vi "AO Engine Testing.vi"(8 "error in (no error)":errorcluster) -> (0 "error out":errorcluster)   [LabVIEW 2009]
doc: "Copyright © 2005, Soliton Technologies.\nAll rights reserved."
uses:
  Controls/SLL DE List of Analog Outputs.ctl
  Controls/SLL DE AO Global Options.ctl
  <vilib>/DAQmx/read.llb/DAQmx Read (Analog DBL 1Chan 1Samp).vi
  <vilib>/DAQmx/create/channels.llb/DAQmx Create Channel (AI-Voltage-Basic).vi
panel:
  in  "stop":bool
  out "x-y":u32=6905
  out "Done?":bool
  out "data":dbl=0.000762939453125 format="%0.2f"
  in  "DAQmx Physical Channel":tag="Dev1/_ao0_vs_aognd"
  in  "AO Option":T1=enum."Write Line"
  in  "List of Analog Outputs":T2
  in  "AO value":dbl=1.0
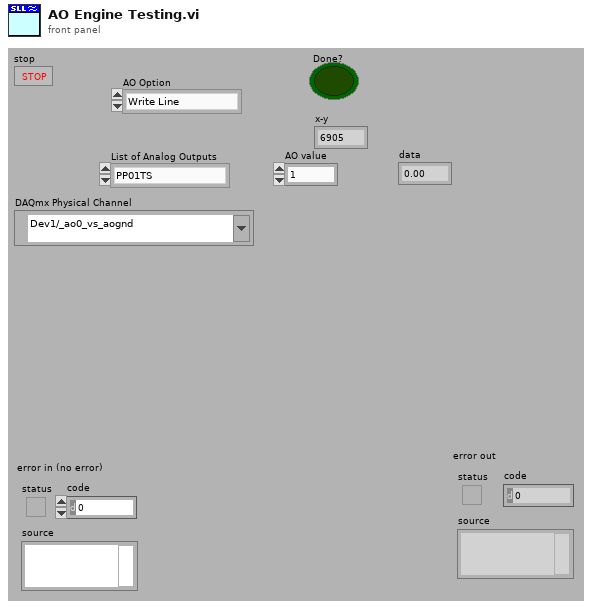
[diagram p1: front panel]
types:
  T1 = typedef "SLL DE AO Global Options.ctl" = enum16{"Init", "Write Line", "Write Array", "Read Line", "Read Array", "Read Full Status", "Restart AO", "Send to Safe Mode", "Stop AO"}
  T2 = typedef "SLL DE List of Analog Outputs.ctl" = enum16{"PP01TS", "PP02TS", "PP03TS"}
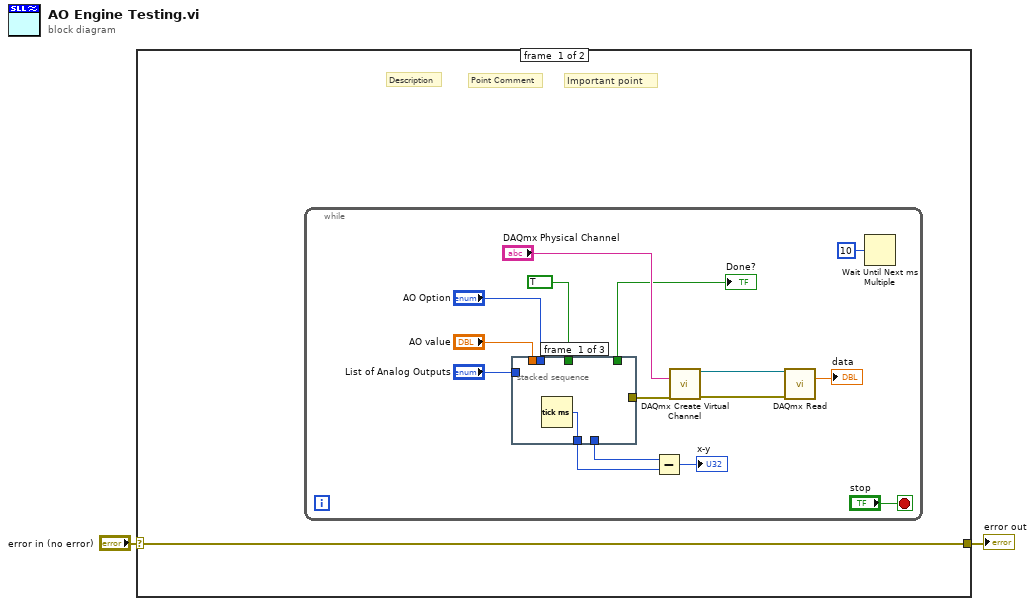
[diagram p0: block diagram]
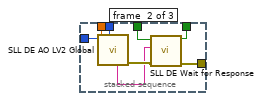
[diagram p2: hidden frame]
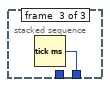
[diagram p3: hidden frame]
diagram:
  n1 = case shown="No Error" "error in (no error)" {
    selector: "error in (no error)" -> [w3 w29]
    tunnel: [w3 w29] -> w1
    frame #0 {
      # "Point Comment"
      # "Important point"
      # "Description"
      n2 = while {
        stop <- "stop" stop-if-true
        n3 = stacked-sequence {
          tunnel: "AO Option" -> [_ w27 _]
          tunnel: "List of Analog Outputs" -> [_ w26 _]
          tunnel: "AO value" -> [_ w25 _]
          tunnel: [_ w23 _] -> w11
          tunnel: [_ w22 _] -> w10
          tunnel: TRUE ("Check Response?") -> [_ w20 _]
          tunnel: [_ _ w28] -> w7
          tunnel: [w19 _ _] -> w8
          frame #0 {
            n4 = Tick Count (ms)() -> (millisecond timer value=w19:u32)
          }
          frame #1 {
            n5 = call "SLL DE AO LV2 Global.vi"("AO Option"=w27, "AO value"=w25, "AO Channel Name"=w26) -> ("error out"=w24:errorcluster, "Element Wrote"=w21:string)  [unwired: 5 in, 2 out]
            n6 = call "SLL DE Wait for Response.vi"("Error In"=w24, "Executed For?"=w21, "Check Response?"=w20) -> ("error out"=w23:errorcluster, "Done?"=w22:bool)  [unwired: 7 in]
          }
          frame #2 {
            n7 = Tick Count (ms)() -> (millisecond timer value=w28:u32)
          }
        }
        "Done?" <- w10
        n8 = Subtract(x=w7, y=w8) -> (x-y=→"x-y":u32)
        n9 = call-poly <vilib>:"DAQmx Create Virtual Channel.vi"("physical channels"="DAQmx Physical Channel", "error in"=w11) -> ("task out"=w14:refnum<k21>, "error out"=w13:errorcluster)  [unwired: 12 in]
        n10 = call-poly <vilib>:"DAQmx Read.vi"("task/channels in"=w14, "error in"=w13) -> ("data"=→"data":dbl)  [unwired: 11 in, 2 out]
        n11 = Wait Until Next ms Multiple(millisecond multiple=u32 10) -> ()  [unwired: 1 out]
      }
    }
    frame #1 {
    }
  }
  "error out" <- w1
